vi "Compute.vi"(8 "error in (no error)":errorcluster, 9 "Data Channels":T3, 10 "x-var":T2(array[cluster]), 11 "Phase in":refnum<class "Phase.lvclass">) -> (0 "error out":errorcluster, 1 "Add'l Data Channels":T3, 3 "Phase out":refnum<class "Phase.lvclass">)   [LabVIEW 2023, in "Phase.lvclass"]
uses:
  Phase.lvclass
  Instruments/Utility Classes/Readable/Data Channels.ctl
  Instruments/Utility Classes/Readable/Data Channel.ctl
  Instruments/Utility Classes/Readable/Data Point.ctl
  Instruments/Utility Classes/Readable/Time.ctl
  Instruments/Utility Classes/Readable/X.ctl
  Instruments/Utility Classes/Readable/Readable.lvclass
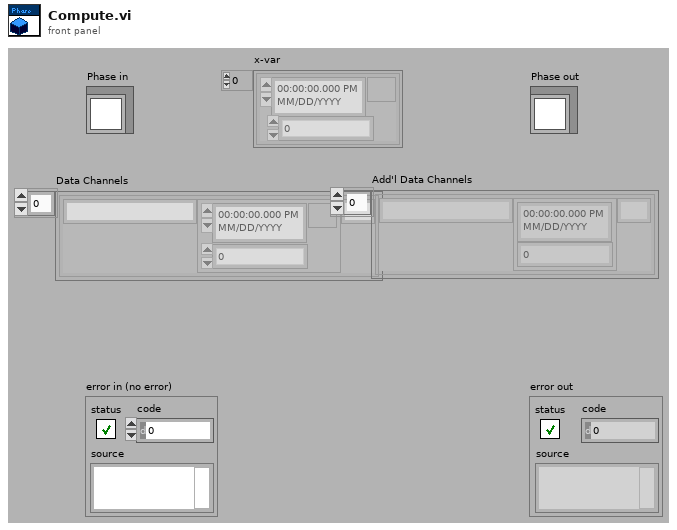
[diagram p1: front panel]
types:
  T1 = typedef "Readable.lvclass/X.ctl" = dbl
  T2 = cluster{"seconds since 1Jan1904":timestamp, "X-Var":T1}[]
  T3 = typedef "Readable.lvclass/Data Channels.ctl" = T4[]
  T4 = typedef "Readable.lvclass/Data Channel.ctl" = cluster{"Name":string, "Data Point":T5, "Unit":string}
  T5 = typedef "Readable.lvclass/Data Point.ctl" = cluster{"t":T6, "x":T1}
  T6 = typedef "Readable.lvclass/Time.ctl" = timestamp
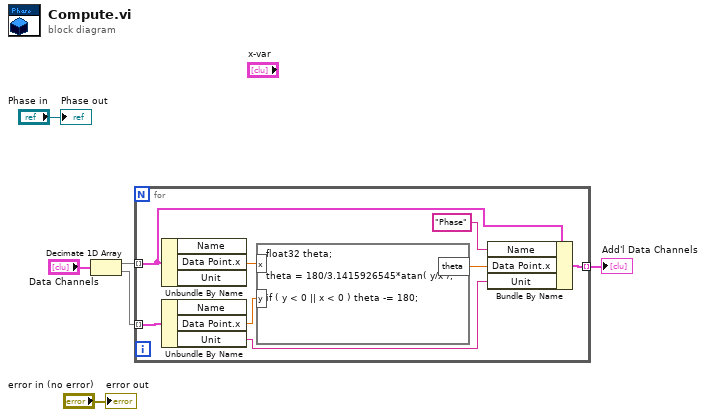
[diagram p0: block diagram]
diagram:
  n1 = Decimate 1D Array("Data Channels") -> (w6:T4[], w5:T4[])
  n2 = for {
    tunnel: w6 -> [w13] mode=indexing
    tunnel: w5 -> [w14] mode=indexing
    tunnel: [w11] -> w3 mode=indexing
    n3 = Unbundle By Name(w13) -> ("Data Point.x"=w8:T1)  [unwired: 2 out]
    n4 = Unbundle By Name(w14) -> ("Data Point.x"=w7:T1, "Unit"=w12:string)  [unwired: 1 out]
    n5 = formula code="float32 theta;\n\ntheta = 180/3.1415926545*atan( y/x );\n\nif ( y < 0 || x < 0 ) theta -= 180;"("x"=w8, "y"=w7) -> ("theta"=w9:sgl)
    n6 = Bundle By Name(cluster=w13, "Name"="Phase" ("format string"), "Data Point.x"=w9, "Unit"=w12) -> (w11:T4)
  }
  "Add'l Data Channels" <- w3
  "error out" <- "error in (no error)"
  "Phase out" <- "Phase in"
